vi "MRC Check Api Version.vi"(8 "error in (no error)":errorcluster, 11 "version":u32) -> (0 "error out":errorcluster, 3 "function return":u8)   [LabVIEW 2026, in "MrcLib.lvlib"]
doc: "MRC_Bool MRC_CheckApiVersion(uint32_t version);"
uses:
  MrcLib.lvlib
  MrcLib.dll
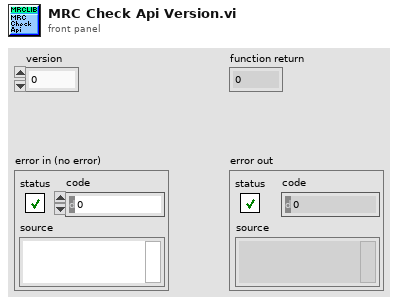
[diagram p1: front panel]
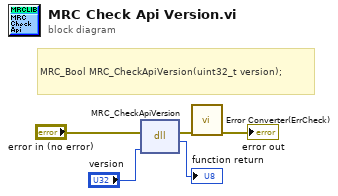
[diagram p0: block diagram]
diagram:
  # "MRC_Bool MRC_CheckApiVersion(uint32_t version);"
  n1 = dll-call lib="MrcLib.*" fn="MRC_CheckApiVersion"(error in="error in (no error)", "version"="version") -> (error out=w2:errorcluster, →"function return":u8)  [unwired: 3 in, 1 out]
  n2 = call "Error Converter(ErrCheck).vi"("error in (no error)"=w2) -> ("error out"=→"error out":errorcluster)  [unwired: 10 in]
